vi "Data Bank (3D).vi"(1 "Action":T1(ring), 7 "2D Data in":dbl[][](array[numeric]), 11 "n":i32) -> (4 "3D Data out":dbl[][][](array[numeric]), 8 "2D Data out":dbl[][](array[numeric]), 15 "Npages":i32)   [LabVIEW 2015]
uses:
  Utility VIs/Array Dimensions (3D).vi
  Utility VIs/Array Dimensions (2D).vi
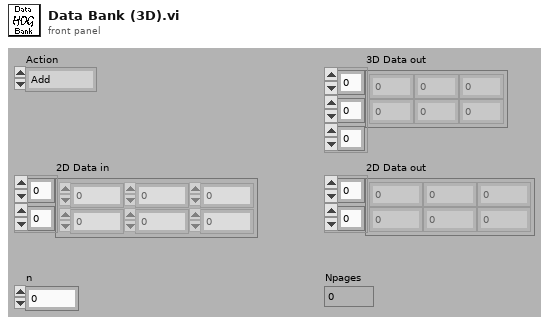
[diagram p1: front panel]
types:
  T1 = enum16{"Add", "Clear", "Read", "Read nth", "Replace nth"}
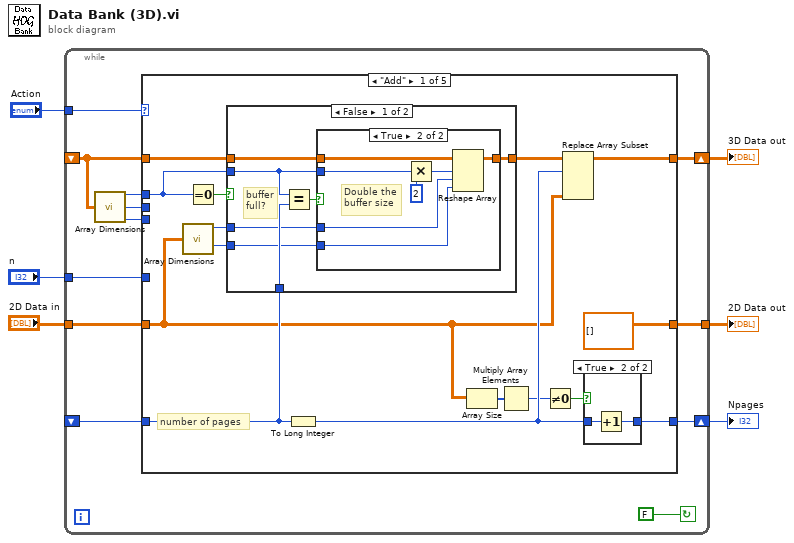
[diagram p0: block diagram]
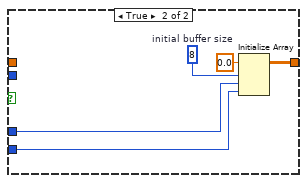
[diagram p4: hidden frame]
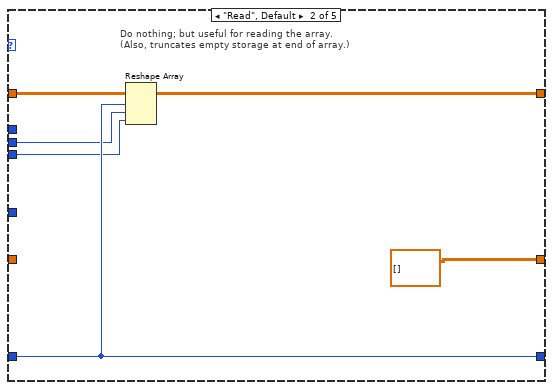
[diagram p5: hidden frame]
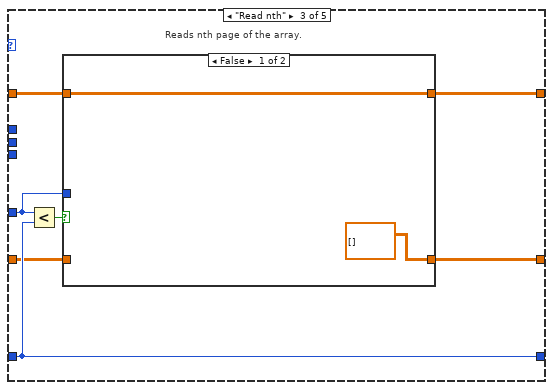
[diagram p6: hidden frame]
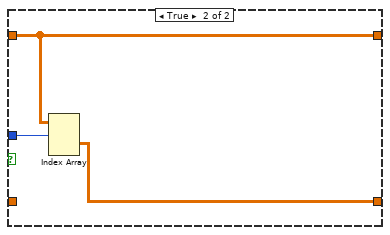
[diagram p7: hidden frame]
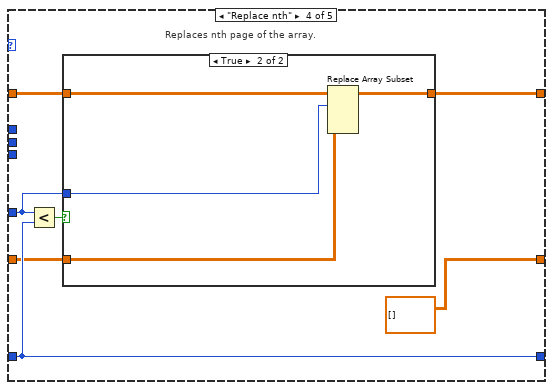
[diagram p8: hidden frame]
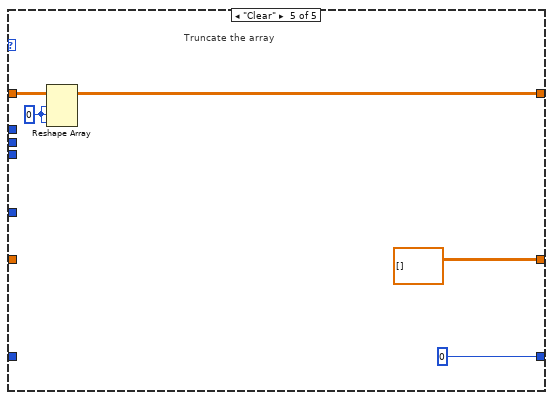
[diagram p10: hidden frame]
diagram:
  n1 = while {
    tunnel: "2D Data in" -> [w14]
    shift-left: _ -> [w16]
    shift-right: [w15] -> w5
    shift-left: _ -> [w10]
    shift-right: [w17] -> w3
    tunnel: "Action" -> [w18]
    tunnel: "n" -> [w12]
    tunnel: [w11] -> w2
    stop <- FALSE continue-if-true
    n2 = call-poly "Array Dimensions.vi"("3D Array"=w10) -> ("# pages"=w7:i32, "# rows"=w9:i32, "# columns"=w8:i32)  [unwired: 12 in]
    n3 = case shown="\"Add\"" w18 {
      tunnel: w10 -> [w31 w61 w67 w79 w91]
      tunnel: [w28 w62 w66 w78 w90] -> w17
      tunnel: w16 -> [w32 w59 w69 w81 _]
      tunnel: [w33 w59 w69 w81 0] -> w15
      tunnel: w14 -> [w21 _ w64 w76 _]
      tunnel: w12 -> [_ _ w65 w77 _]
      tunnel: [dbl[][] [] ("2D Data in") dbl[][] [] ("2D Data in") w63 dbl[][] [] ("2D Data in") dbl[][] [] ("2D Data in")] -> w11
      tunnel: w7 -> [w25 _ _ _ _]
      tunnel: w9 -> [_ w58 _ _ _]
      tunnel: w8 -> [_ w57 _ _ _]
      frame "Add" {
        # "number of pages"
        n4 = call-poly "Array Dimensions.vi"("2D Array"=w21) -> ("# rows"=w22:i32, "# columns"=w23:i32)  [unwired: 13 in]
        n5 = Equal To 0?(x=w25) -> (x = 0?=w26:bool)
        n6 = case shown="False" w26 {
          tunnel: w32 -> [w42 _]
          tunnel: w31 -> [w41 _]
          tunnel: [w40 w52] -> w29
          tunnel: w25 -> [w39 _]
          tunnel: w22 -> [w38 w54]
          tunnel: w23 -> [w37 w53]
          frame False {
            # "buffer\nfull?"
            n7 = Equal?(x=w39, y=w42) -> (x = y?=w43:bool)
            n8 = case shown="True" w43 {
              tunnel: w41 -> [w44 w45]
              tunnel: [w44 w51] -> w40
              tunnel: w39 -> [_ w49]
              tunnel: w38 -> [_ w47]
              tunnel: w37 -> [_ w46]
              frame False {
              }
              frame True {
                # "Double the\nbuffer size"
                n9 = Multiply(x=w49, y=2) -> (x*y=w48:i32)
                n10 = Reshape Array(w45, w48, w47, w46) -> (w51:dbl[][][])
              }
            }
          }
          frame True {
            w56 = 8  # initial buffer size
            n11 = Initialize Array(0.0 ("element"), w56, w54, w53) -> (w52:dbl[][][])
          }
        }
        n12 = To Long Integer(number=w32) -> (32bit integer=w27:i32)
        n13 = Array Size(array=w21) -> (size(s)=w20:i32[])
        n14 = Multiply Array Elements(1:w20) -> (0:w19:i32)
        n15 = Not Equal To 0?(x=w19) -> (x != 0?=w24:bool)
        n16 = Replace Array Subset(array=w29, new element=w21, index (dim 0)=w27) -> (w28:dbl[][][])  [unwired: 2 in]
        n17 = case shown="True" w24 {
          tunnel: [w34 w36] -> w33
          tunnel: w27 -> [w34 w35]
          frame False {
          }
          frame True {
            n18 = Increment(x=w35) -> (x+1=w36:i32)
          }
        }
      }
      frame "Read", Default {
        # "Do nothing; but useful for reading the array.\n(Also, truncates empty storage at end of array.)"
        n19 = Reshape Array(w61, w59, w58, w57) -> (w62:dbl[][][])
      }
      frame "Read nth" {
        # "Reads nth page of the array."
        n20 = Less?(x=w65, y=w69) -> (x < y?=w68:bool)
        n21 = case shown="False" w68 {
          tunnel: w67 -> [w71 w73]
          tunnel: [w71 w73] -> w66
          tunnel: w65 -> [_ w72]
          tunnel: w64 -> [_ _]
          tunnel: [dbl[][] [] ("Modified 2D Array") w74] -> w63
          frame False {
          }
          frame True {
            n22 = Index Array(array=w73, index (dim 0)=w72) -> (element=w74:dbl[][])  [unwired: 2 in]
          }
        }
      }
      frame "Replace nth" {
        # "Replaces nth page of the array."
        n23 = Less?(x=w77, y=w81) -> (x < y?=w80:bool)
        n24 = case shown="True" w80 {
          tunnel: w79 -> [w82 w86]
          tunnel: [w82 w84] -> w78
          tunnel: w77 -> [_ w83]
          tunnel: w76 -> [_ w85]
          frame False {
          }
          frame True {
            n25 = Replace Array Subset(array=w86, new element=w85, index (dim 0)=w83) -> (w84:dbl[][][])  [unwired: 2 in]
          }
        }
      }
      frame "Clear" {
        w88 = 0
        # "Truncate the array"
        n26 = Reshape Array(w91, w88, w88, w88) -> (w90:dbl[][][])
      }
    }
  }
  "Npages" <- w5
  "3D Data out" <- w3
  "2D Data out" <- w2
